vi "rawpower2totalprad.vi"(1 "SampleTime":sgl=0.0032, 3 "width":i32=1, 4 "threshold":dbl=0.00012, 8 "Pre-start time (ms) of\nDAQ":i32=10000, 9 "AddOnTime":sgl=5.0, 10 "samples to exclude":u32=1000, 11 "kbolott_and_volume":dbl[][](array[numeric])=[[1e-05, 1e-05], [9.8364458e-05, 1.8160732], [0.00029863964, 770.25441], [0.00053910452, 1653.5432], [0.00071569496, 2554.7619], [0.00083348142, 3356.1809], [0.00092645429, 4021.9678], [0.00099241932, 4570.4466], [0.0010332482, 4989.6792], [0.0010552469, 5170.4882], [0.0010669981, 5192.5645], [0.001071534, 5152.6222], [0.0010766644, 5109.6704], [0.0010841289, 5094.9972], [0.0010884845, 5078.237], [0.0010888843, 5058.9416], [0.0010882289, 5056.581], [0.0010872861, 5078.1684], [0.0010832221, 5096.5196], [0.0010760805, 5113.7904], [0.0010685167, 5141.4566], [0.0010644166, 5189.7831], [0.0010539441, 5182.7365], [0.0010337779, 5034.6928], [0.00098716411, 4625.8518], [0.00091599422, 4090.3707], [0.00082376071, 3438.9665], [0.00070194108, 2659.5109], [0.00051785958, 1753.3355], [0.00030745544, 937.82125], [0.00014081292, 59.55205], [1e-05, 1e-05], [0.0, 0.0], [0.0, 0.0], [0.0, 0.0], [0.0, 0.0], [0.0, 0.0], [0.0, 0.0], [0.0, 0.0], [0.0, 0.0], [0.0, 0.0], [0.0, 0.0], [0.0, 0.0], [0.0, 0.0], [0.0, 0.0], [0.0, 0.0], [0.0, 0.0], [0.0, 0.0], [0.0019134875, 3474.3085], [0.0020594744, 3690.1455], [0.002175929, 3861.3028], [0.0022530617, 3956.5918], [0.0023492529, 4057.9903], [0.0024581424, 4205.0841], [0.0025383764, 4324.9746], [0.0025876415, 4417.9525], [0.0026676725, 4566.0612], [0.0027635964, 4770.6296], [0.0028188521, 4914.295], [0.0028263806, 4970.0105], [0.0028491244, 5014.7926], [0.0028762033, 5060.279], [0.0028430703, 4969.1072], [0.0027058578, 4592.2853], [0.0019047772, 4936.5706], [0.0023594746, 6388.5028], [0.0025094117, 6336.5413], [0.002569351, 6048.9284], [0.0026367277, 5794.3031], [0.002714522, 5668.1597], [0.0027530637, 5505.217], [0.0027520905, 5312.6378], [0.0027781484, 5183.8321], [0.0028283925, 5165.5044], [0.0028425709, 5118.655], [0.00281436, 5016.5122], [0.0027996491, 4909.784], [0.0027993913, 4845.125], [0.0027603692, 4728.4661], [0.0026886073, 4585.7454], [0.0026437627, 4495.4419], [0.0026242501, 4486.7206], [0.0025685332, 4434.986], [0.0024747416, 4324.8822], [0.0023915919, 4209.8149], [0.002319616, 4111.844], [0.0022042921, 3923.4955], [0.0020485146, 3644.5259], [0.0024033884, 3597.1969], [0.002066694, 2566.1598], [0.0017718795, 1878.4004], [0.0015136288, 1414.3006], [0.0013043692, 1094.5581], [0.0011378765, 882.65731], [0.00097324167, 712.97006], [0.00080739571, 571.52867], [0.0, 0.0], [0.0, 0.0], [0.0, 0.0], [0.0, 0.0], [0.0, 0.0], [0.0, 0.0], [0.0, 0.0], [0.0, 0.0], [0.0, 0.0], [0.0, 0.0], [0.0, 0.0], [0.0, 0.0], [0.0, 0.0], [0.0, 0.0], [0.0, 0.0], [0.0, 0.0], [0.0, 0.0], [0.0, 0.0], [0.0, 0.0], [0.0, 0.0], [0.0, 0.0], [0.0, 0.0], [0.0, 0.0], [0.0, 0.0], [0.0, 0.0], [0.0, 0.0], [0.0, 0.0], [0.0, 0.0], [0.0, 0.0], [0.0, 0.0], [0.0, 0.0], [0.0, 0.0]], 12 "No. of Samples\n[TOA / Sample Rate]":i32=8829, 13 "tau_fact":dbl[](array[numeric])=[0.9942754325698635, 0.9942874264772165, 0.9945323434853295, 0.9944942634351588, 0.9943224506450672, 0.9943408937418631, 0.995821993302933, 0.9945771384409823, 0.9944620036742867, 0.9944762183578384, 0.9939064850392964, 0.9942348416823442, 0.9941481394691951, 0.9939736217416081, 0.9940920651258721, 0.9938858383903332, 0.9946231806379121, 0.9946794273486279, 0.9945386493082798, 0.9945088068622799, 0.9885887214081416, 0.9944821982358365, 0.9942590170035959, 0.9943949158017914, 0.9944259674033434, 0.9942557134338033, 0.9943682303140012, 0.9944129847299683, 0.9937053838258036, 0.9937063363597569, 0.9937961958887874, 0.993777190579244, 0.9967727911662049, 0.9954284436124313, 0.9947198089384633, 0.9947945758851272, 0.992855835614686, 0.9951259961796087, 0.9915396916800793, 0.9938777213378227, 0.9925620075631091, 0.9939808571119726, 0.9953730857234031, 0.9949446485350009, 0.9951693651989406, 0.9938965230094928, 0.9939251148981592, 0.993919756464684, 0.9955634864440348, 0.9965442790473252, 0.9958326248057368, 0.9959297989255841, 0.9946741668106229, 0.9961317432538527, 0.9940816674176194, 0.9956134846505059, 0.994696761237249, 0.9956489327005682, 0.9957202726127232, 0.9952614295331398, 0.9953602706677246, 0.9943075252732968, 0.99446916653835, 0.9944158295695202, 0.9942767772483964, 0.9941050695859821, 0.9944374591927472, 0.9945090337805454, 0.994559907934673, 0.9945848227562215, 0.9948370294812288, 0.9946407805595008, 0.9947163757511401, 0.9944559864420973, 0.994448676943994, 0.9945138262559567, 0.9946225671933909, 0.9946033931105569, 0.9945303195379069, 0.9943576342591244, 0.9939005664775309, 0.993829355141712, 0.9940758603249683, 0.9945212190107237, 0.9945653472775302, 0.9944883825084508, 0.9944285415381326, 0.9969718967619399, 0.9934533430051062, 0.9934476065516122, 0.994137584128452, 0.9939183969854989, 0.9929544573919961, 0.9927976688292449, 0.9926525324439995, 0.9925179780752803, 0.993697881831798, 0.9938832006928247, 0.9939451412935264, 1.0, 0.9934735935885004, 0.9936498588825847, 0.9936377263535082, 0.9938649606619758, 0.9927081189806816, 0.9928561967168806, 0.9930023684194763, 0.9930998249399461, 0.9931265778529161, 0.9931539659381708, 0.9932420399385089, 1.0, 0.9931786270549593, 1.0, 1.0, 1.0, 1.0, 1.0, 1.0, 1.0, 1.0, 1.0, 1.0, 1.0, 1.0, 1.0, 1.0, 1.0], 15 "F_ch":dbl[](array[numeric])=[0.41946313361925236, 0.41267288435379323, 0.4242513967796445, 0.4168638482034789, 0.41940297094410406, 0.41277199910121876, 0.5005048325232518, 0.41804357116097796, 0.4263914266029813, 0.42960951092847915, 0.390161915811526, 0.40903209292753795, 0.4178724636706656, 0.40639561524491535, 0.4168972961680756, 0.4081753936316892, 0.4308482203292378, 0.42985423214074037, 0.4219523533476951, 0.42368590442341997, 0.14968177217291742, 0.4163100359962662, 0.4023134454260441, 0.414083420090156, 0.4104404162383056, 0.40109746288400294, 0.4118376955811143, 0.4106810858926003, 0.4024662767215043, 0.39776761041402614, 0.39988820944073605, 0.3960937680653605, 0.39631376832177734, 0.46359628762328325, 0.4330664870101722, 0.42809053434855326, 0.3663794753981563, 0.4515112216941263, 0.32097119732923274, 0.38596625816052027, 0.35592992953912717, 0.3967614343688723, 0.4769395376117402, 0.4603968175127216, 0.45645057575669823, 0.40983050619896044, 0.41762784967370237, 0.4195235233012393, 0.4869668482151368, 0.5451176818983113, 0.4981002466254468, 0.5025919311483945, 0.4408139623514431, 0.5086015118188133, 0.4212525350361159, 0.489548299707763, 0.44280968589083947, 0.4733195391787026, 0.48968023906864, 0.46123705868954207, 0.48585880384966634, 0.43109305912935353, 0.42964432162914334, 0.43379373132681903, 0.4103150055137274, 0.41637546628976474, 0.4240718501347476, 0.43097541489804153, 0.42854727670203413, 0.43071258286250785, 0.4538231011436137, 0.43842591900842043, 0.44773109787963017, 0.43813274820972226, 0.4477786314686775, 0.43083627933543217, 0.4448007784686704, 0.4463858689900978, 0.44471759411780265, 0.43905527786878207, 0.40988850494900064, 0.4042286595549796, 0.4210125779131261, 0.42523385782519874, 0.43930897084124976, 0.4317134422486339, 0.42503793161390413, 0.5866703715028357, 0.3713420175081803, 0.3729221791024955, 0.421847369908469, 0.4038171530405619, 0.3723947010396081, 0.36905241334809796, 0.365027355646126, 0.35883096352560634, 0.38453723852279414, 0.3908590433215044, 0.3942344477458136, -inf, 0.37872098293573886, 0.38823921546406664, 0.38647066465095736, 0.4010630278464888, 0.3699009376238012, 0.37440275442115767, 0.378492662918438, 0.37713022559389764, 0.375270284145916, 0.37421667685537685, 0.3729410641899398, inf, 0.367989869633843, -inf, -inf, -inf, -inf, -inf, inf, -inf, -inf, -inf, -inf, inf, inf, inf, -inf, inf], 17 "TauM":dbl[](array[numeric])=[0.10247326273143675, 0.10385139756960429, 0.10373232144795708, 0.10311875959492485, 0.1040387663981229, 0.1046650716638566, 0.10127197371489062, 0.10433939668939028, 0.09961240211936159, 0.10113688577012743, 0.09820100289764892, 0.10095901838579123, 0.10145991266213297, 0.10133898562095205, 0.10130127833216106, 0.09956334469474118, 0.10358378126227558, 0.1033444650149854, 0.10368122845865657, 0.1024629201687842, 0.10726822954303422, 0.10182022977214773, 0.10234341921814957, 0.10309722284273504, 0.1042952251760315, 0.10251907726247211, 0.10376892017069193, 0.10390613836510422, 0.10393962152806514, 0.10278682866750612, 0.1029066416867304, 0.102809145991027, 0.10885131092677319, 0.09862497604372066, 0.10044854636642224, 0.1011397796494332, 0.10002902352125999, 0.09964990042145319, 0.10015936689391987, 0.10006472096945454, 0.09839726301474191, 0.0989699304142558, 0.1002391552504395, 0.10013350870556857, 0.10080436633835735, 0.09779852218595043, 0.09742571115181148, 0.09710433370493086, 0.10444501045101653, 0.1003366401072974, 0.10437315691375147, 0.10384291417884778, 0.10124021541103015, 0.10550745222701648, 0.1035137865735804, 0.10352859881892808, 0.1012417667717822, 0.1059159267079176, 0.10317764912629153, 0.10345604684447908, 0.1049337703539443, 0.10334536377187596, 0.1011439242990685, 0.10281039287381427, 0.10222071286894058, 0.10128943771143158, 0.10126644136767568, 0.10213051552429299, 0.10166794227392674, 0.10164755793457868, 0.10028065773083647, 0.1039274155284877, 0.10062166309448936, 0.10100667896022858, 0.10122793031614634, 0.1020869722455638, 0.10086834901007827, 0.10107073060568635, 0.10100593381229647, 0.1013148799331511, 0.10336010473304796, 0.104020047148851, 0.10319519163947051, 0.1023647743297228, 0.10121262984849082, 0.10131571623308212, 0.10129251089534078, 0.10505043416568437, 0.10066202738446095, 0.10001990246198598, 0.10320829246582676, 0.10342094956544687, 0.10072458787609094, 0.10113661913958252, 0.10213104126735983, 0.10141193462449195, 0.10097352152629059, 0.1005352087055146, 0.09991412160243203, 0.0, 0.09971962753116924, 0.10038664478845472, 0.0996831725438015, 0.0987164166127979, 0.10070743969491262, 0.10083769719722958, 0.09991070137880578, 0.09976037466686079, 0.09975950391708734, 0.0997863315853558, 0.09952725945462769, 0.0, 0.09982037400508142, 0.0, 0.0, 0.0, 0.0, 0.0, 0.0, 0.0, 0.0, 0.0, 0.0, 0.0, 0.0, 0.0, 0.0, 0.0] format="%10.4f", 19 "RawArray":sgl[][](array[numeric])=array128x7829[1002112 elements]) -> (16 "corrected voltage array":dbl[][](array[numeric]), 18 "AdjustedPower":dbl[][](array[numeric]), 22 "P_rad HBC [MW]":dbl[](array[numeric]), 23 "P_rad VBC [MW]":dbl[](array[numeric]))   [LabVIEW 2014]
uses:
  <vilib>/Analysis/baseanly.llb/Mean (DBL).vi
  <vilib>/Analysis/3filter.llb/FIR Filter (DBL).vi
  <vilib>/Analysis/NI_AALBase.lvlib
  <vilib>/Analysis/NI_AALPro.lvlib
  <vilib>/Analysis/3filter.llb/Savitzky-Golay Filter (DBL).vi
panel:
  out "Time":dbl[](array[numeric])
  out "ECRH OFF SAMPLE":i64
  out "empty sample array":dbl[](array[numeric])
  out "ECRH ON SAMPLE":i64=2156
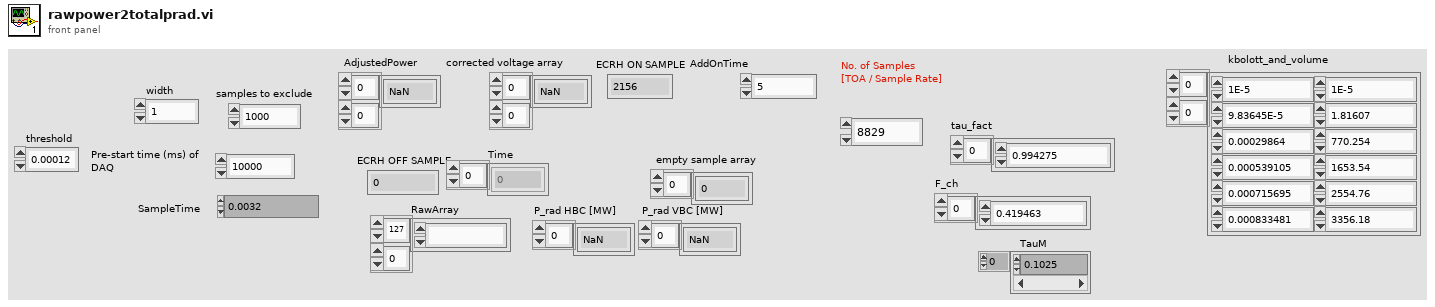
[diagram p1: front panel]
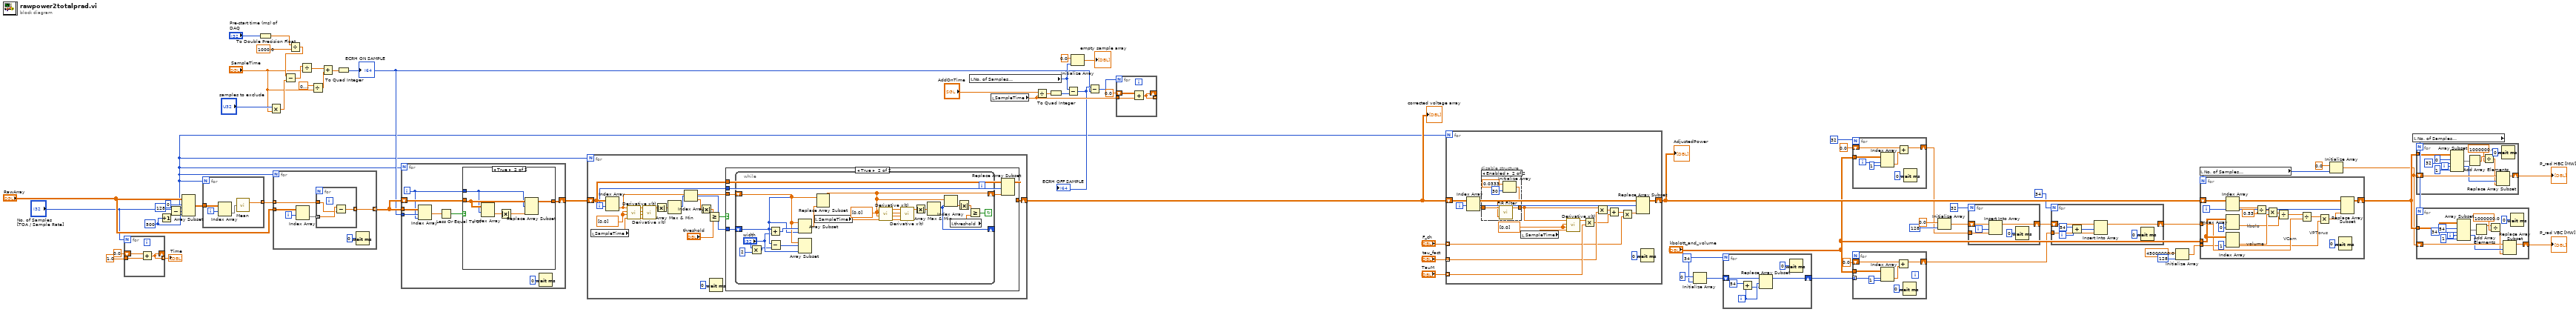
[diagram p0: block diagram]
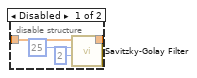
[diagram p3: hidden frame]
diagram:
  w36 = 34
  w2 = 128 ("length")
  w11 = 500 ("y")
  n1 = for {
    N: "No. of Samples\n[TOA / Sample Rate]" -> [_]
    tunnel: [w72] -> w4 mode=indexing
    shift-right: [w72] -> _
    shift-left: 0.0 -> [w71]
    tunnel: sgl 1.0 ("SampleTime") -> [w70]
    n2 = Add(x=w71, y=w70) -> (x+y=w72:dbl)
  }
  "Time" <- w4
  n3 = Increment(x=w11) -> (x+1=w10:i32)
  n4 = Subtract(x="No. of Samples\n[TOA / Sample Rate]", y=w10) -> (x-y=w69:i32)
  n5 = Array Subset(array="RawArray", index (row)=0 ("index"), length (row)=w2, index (col)=w69, length (col)=w11) -> (w67:sgl[][])
  n6 = for {
    N: w2 -> [_]
    tunnel: w67 -> [w74]
    tunnel: [w76] -> w66 mode=indexing
    i -> [w73]
    n7 = Index Array(array=w74, index (row)=w73) -> (element=w75:sgl[])  [unwired: 1 in]
    n8 = call-poly <vilib>:"Mean.vi"("X"=w75) -> ("mean"=w76:dbl)  [unwired: 1 out]
  }
  n9 = To Double Precision Float(number="Pre-start time (ms) of\nDAQ") -> (double precision float=w61:dbl)
  n10 = Multiply(x="samples to exclude", y="SampleTime") -> (x*y=w63:sgl)
  n11 = for {
    N: w2 -> [_]
    tunnel: w66 -> [w80] mode=indexing
    tunnel: "RawArray" -> [w82]
    tunnel: [w78] -> w53 mode=indexing
    i -> [w81]
    n12 = Index Array(array=w82, index (row)=w81) -> (element=w79:sgl[])  [unwired: 1 in]
    n13 = for {
      tunnel: w79 -> [w85] mode=indexing
      tunnel: w80 -> [w84]
      tunnel: [w83] -> w78 mode=indexing
      n14 = Subtract(x=w85, y=w84) -> (x-y=w83:dbl)
    }
    n15 = Wait (ms)(milliseconds to wait=u32 0) -> ()  [unwired: 1 out]
  }
  n16 = Divide(x=w61, y=1000.0) -> (x/y=w59:dbl)
  n17 = Subtract(x=w59, y=w63) -> (x-y=w62:dbl)
  n18 = Divide(x=w62, y="SampleTime") -> (x/y=w58:dbl)
  n19 = Divide(x=sgl 0.1, y="SampleTime") -> (x/y=w54:sgl)
  n20 = Add(x=w58, y=w54) -> (x+y=w57:dbl)
  n21 = To Quad Integer(1:w57) -> (0:w3:i64)
  "ECRH ON SAMPLE" <- w3
  n22 = for {
    N: w2 -> [_]
    tunnel: w53 -> [w93]
    tunnel: w3 -> [w92]
    shift-right: [w87] -> w8
    shift-left: w53 -> [w89]
    i -> [w88]
    n23 = Index Array(array=w93, index (row)=w92, index (col)=w88) -> (element=w91:dbl)
    n24 = Less Or Equal To 0?(x=w91) -> (x <= 0?=w90:bool)
    n25 = case shown="True" w90 {
      tunnel: w89 -> [w94 w99]
      tunnel: w88 -> [_ w98]
      tunnel: [w94 w97] -> w87
      frame False {
      }
      frame True {
        n26 = Index Array(array=w99, index (row)=w98) -> (element=w96:dbl[])  [unwired: 1 in]
        n27 = Absolute Value(x=w96) -> (abs(x)=w95:dbl[])
        n28 = Replace Array Subset(array=w99, new element=w95, index (row)=w98) -> (w97:dbl[][])  [unwired: 1 in]
      }
    }
    n29 = Wait (ms)(milliseconds to wait=u32 0) -> ()  [unwired: 1 out]
  }
  n30 = for {
    N: w2 -> [_]
    shift-right: [w101] -> w7
    shift-left: w8 -> [w108]
    i -> [w100]
    w113 = dbl[] [0.0] ("Initial Condition")
    n31 = local read "SampleTime"() -> (w112:sgl)
    n32 = Index Array(array=w108, index (row)=w100) -> (element=w102:dbl[])  [unwired: 1 in]
    n33 = call <vilib>:"Derivative x(t).vi"("dt"=w112, "Final Condition"=w113, "Initial Condition"=w113, "X"=w102) -> ("dX/dt"=w114:dbl[])  [unwired: 6 in, 1 out]
    n34 = call <vilib>:"Derivative x(t).vi"("dt"=w112, "Final Condition"=w113, "Initial Condition"=w113, "X"=w114) -> ("dX/dt"=w111:dbl[])  [unwired: 6 in, 1 out]
    n35 = Absolute Value(x=w111) -> (abs(x)=w103:dbl[])
    n36 = Array Max & Min(array=w103) -> (max index (indices)=w107:i32)  [unwired: 3 out]
    n37 = Index Array(array=w102, index=w107) -> (element=w106:dbl)
    n38 = Absolute Value(x=w106) -> (abs(x)=w105:dbl)
    n39 = Greater Or Equal?(x=w105, y="threshold") -> (x >= y?=w109:bool)
    n40 = Wait (ms)(milliseconds to wait=u32 0) -> ()  [unwired: 1 out]
    n41 = case shown="True" w109 {
      tunnel: w102 -> [_ w121]
      tunnel: w100 -> [_ w116]
      tunnel: w108 -> [w115 w119]
      tunnel: [w115 w118] -> w101
      tunnel: w107 -> [_ w120]
      frame False {
      }
      frame True {
        n42 = while {
          shift-right: [w122] -> w117
          shift-left: w121 -> [w137]
          shift-right: [w126] -> _
          shift-left: w120 -> [w136]
          stop <- w127 continue-if-true
          w134 = dbl[] [0.0] ("Initial Condition")
          n43 = Multiply(x="width", y=2) -> (x*y=w123:i32)
          n44 = Add(x=w136, y="width") -> (x+y=w138:i32)
          n45 = Subtract(x=w136, y=w123) -> (x-y=w139:i32)
          n46 = Array Subset(array=w137, index=w138, length=w136) -> (w135:dbl[])
          n47 = Array Subset(array=w137, index=w139, length="width") -> ()  [unwired: 1 out]
          n48 = local read "SampleTime"() -> (w140:sgl)
          n49 = Replace Array Subset(array=w137, new element=w135, index=w136) -> (w122:dbl[])
          n50 = call <vilib>:"Derivative x(t).vi"("dt"=w140, "Final Condition"=w134, "Initial Condition"=w134, "X"=w122) -> ("dX/dt"=w133:dbl[])  [unwired: 6 in, 1 out]
          n51 = call <vilib>:"Derivative x(t).vi"("dt"=w140, "Final Condition"=w134, "Initial Condition"=w134, "X"=w133) -> ("dX/dt"=w131:dbl[])  [unwired: 6 in, 1 out]
          n52 = Absolute Value(x=w131) -> (abs(x)=w132:dbl[])
          n53 = Array Max & Min(array=w132) -> (max index (indices)=w126:i32)  [unwired: 3 out]
          n54 = Index Array(array=w122, index=w126) -> (element=w130:dbl)
          n55 = local read "threshold"() -> (w128:dbl)
          n56 = Absolute Value(x=w130) -> (abs(x)=w129:dbl)
          n57 = Greater Or Equal?(x=w129, y=w128) -> (x >= y?=w127:bool)
        }
        n58 = Replace Array Subset(array=w119, new element=w117, index (row)=w116) -> (w118:dbl[][])  [unwired: 1 in]
      }
    }
  }
  "corrected voltage array" <- w7
  n59 = local read "No. of Samples\n[TOA / Sample Rate]"() -> (w44:i32)
  n60 = local read "SampleTime"() -> (w48:sgl)
  n61 = Divide(x="AddOnTime", y=w48) -> (x/y=w51:sgl)
  n62 = To Quad Integer(1:w51) -> (0:w50:i64)
  n63 = Subtract(x=w44, y=w50) -> (x-y=w46:i64)
  "ECRH OFF SAMPLE" <- w46
  n64 = Initialize Array(0.0 ("element"), w44) -> (→"empty sample array":dbl[])
  n65 = Subtract(x=w46, y=w3) -> (x-y=w47:i64)
  n66 = for {
    N: w47 -> [_]
    tunnel: [w143] -> _ mode=indexing
    shift-right: [w143] -> _
    shift-left: 0.0 -> [w142]
    tunnel: w48 -> [w141]
    n67 = Add(x=w142, y=w141) -> (x+y=w143:dbl)
  }
  n68 = for {
    N: w2 -> [_]
    shift-right: [w157] -> w39
    shift-left: w7 -> [w156]
    tunnel: "F_ch" -> [w149] mode=indexing
    tunnel: "tau_fact" -> [w153] mode=indexing
    tunnel: "TauM" -> [w154] mode=indexing
    i -> [w155]
    w159 = dbl[] [0.0] ("Initial Condition")
    n69 = Index Array(array=w156, index (row)=w155) -> (element=w147:dbl[])  [unwired: 1 in]
    n70 = disable-structure shown="Enabled" {
      disable-tunnel: w147 -> [w161 w167]
      disable-tunnel: [w160 w166] -> w145
      frame Disabled {
        n71 = call-poly <vilib>:"Savitzky-Golay Filter.vi"("polynomial order"=2, "side points"=25, "X"=w161) -> ("Filtered X"=w160:dbl[])  [unwired: 7 in, 1 out]
      }
      frame Enabled {
        n72 = Initialize Array(0.0333 ("element"), 30 ("dimension size")) -> (w164:dbl[])
        n73 = call-poly <vilib>:"FIR Filter.vi"("FIR Coefficients"=w164, "X"=w167) -> ("Filtered X"=w166:dbl[])  [unwired: 2 in, 1 out]
      }
    }
    n74 = local read "SampleTime"() -> (w158:sgl)
    n75 = call <vilib>:"Derivative x(t).vi"("dt"=w158, "Final Condition"=w159, "Initial Condition"=w159, "X"=w145) -> ("dX/dt"=w146:dbl[])  [unwired: 6 in, 1 out]
    n76 = Multiply(x=w146, y=w154) -> (x*y=w151:dbl[])
    n77 = Multiply(x=w145, y=w153) -> (x*y=w152:dbl[])
    n78 = Add(x=w152, y=w151) -> (x+y=w150:dbl[])
    n79 = Multiply(x=w150, y=w149) -> (x*y=w148:dbl[])
    n80 = Replace Array Subset(array=w156, new element=w148, index (row)=w155) -> (w157:dbl[][])  [unwired: 1 in]
    n81 = Wait (ms)(milliseconds to wait=u32 0) -> ()  [unwired: 1 out]
  }
  "AdjustedPower" <- w39
  n82 = Initialize Array(0, w36) -> (w35:i32[])
  n83 = for {
    N: w36 -> [_]
    shift-right: [w170] -> w34
    shift-left: w35 -> [w171]
    i -> [w174]
    n84 = Add(x=54, y=w174) -> (x+y=w172:i32)
    n85 = Replace Array Subset(array=w171, new element=w172, index=w174) -> (w170:i32[])
    n86 = Wait (ms)(milliseconds to wait=u32 0) -> ()  [unwired: 1 out]
  }
  n87 = for {
    tunnel: "kbolott_and_volume" -> [w181]
    shift-right: [w177] -> w25
    shift-left: 0.0 ("V_Cam") -> [w178]
    tunnel: w34 -> [w176] mode=indexing
    n88 = Index Array(array=w181, index (row)=w176, index (col)=1 ("disabled index (col)")) -> (element=w180:dbl)
    n89 = Add(x=w178, y=w180) -> (x+y=w177:dbl)
    n90 = Wait (ms)(milliseconds to wait=u32 0) -> ()  [unwired: 1 out]
  }
  n91 = for {
    N: 32 -> [_]
    tunnel: "kbolott_and_volume" -> [w188]
    shift-right: [w184] -> w27
    shift-left: 0.0 ("V_Cam") -> [w185]
    i -> [w183]
    n92 = Index Array(array=w188, index (row)=w183, index (col)=1 ("disabled index (col)")) -> (element=w187:dbl)
    n93 = Add(x=w185, y=w187) -> (x+y=w184:dbl)
    n94 = Wait (ms)(milliseconds to wait=u32 0) -> ()  [unwired: 1 out]
  }
  n95 = Initialize Array(0.0 ("element"), 128 ("dimension size")) -> (w29:dbl[])
  n96 = for {
    N: 32 -> [_]
    shift-right: [w190] -> w26
    shift-left: w29 -> [w193]
    tunnel: w27 -> [w191]
    i -> [w192]
    n97 = Insert Into Array(array=w193, index=w192, new element=w191) -> (w190:dbl[])
    n98 = Wait (ms)(milliseconds to wait=u32 0) -> ()  [unwired: 1 out]
  }
  n99 = for {
    N: 34 -> [_]
    shift-right: [w195] -> w24
    shift-left: w26 -> [w198]
    tunnel: w25 -> [w196]
    i -> [w199]
    n100 = Add(x=54, y=w199) -> (x+y=w197:i32)
    n101 = Insert Into Array(array=w198, index=w197, new element=w196) -> (w195:dbl[])
    n102 = Wait (ms)(milliseconds to wait=u32 0) -> ()  [unwired: 1 out]
  }
  n103 = Initialize Array(45000000.0 ("element"), 128 ("dimension size")) -> (w21:dbl[])
  n104 = local read "No. of Samples\n[TOA / Sample Rate]"() -> (w18:i32)
  n105 = for {
    N: w18 -> [_]
    tunnel: "kbolott_and_volume" -> [w218]
    tunnel: w24 -> [w208]
    tunnel: w21 -> [w206]
    shift-right: [w202] -> w20
    shift-left: w39 -> [w205]
    i -> [w204]
    # "VPTorus"
    # "VCam"
    # "kbolo"
    # "volume"
    n106 = Index Array(array=w205, index (col)=w204) -> (element=w215:dbl[])  [unwired: 1 in]
    n107 = Index Array(array=w218, index (col)=0 ("disabled index (col)")) -> (element=w210:dbl[])  [unwired: 1 in]
    n108 = Index Array(array=w218, index (col)=1 ("disabled index (col)")) -> (element=w212:dbl[])  [unwired: 1 in]
    n109 = Divide(x=w215, y=0.53) -> (x/y=w213:dbl[])
    n110 = Multiply(x=w213, y=w212) -> (x*y=w211:dbl[])
    n111 = Divide(x=w211, y=w210) -> (x/y=w209:dbl[])
    n112 = Divide(x=w209, y=w208) -> (x/y=w207:dbl[])
    n113 = Multiply(x=w207, y=w206) -> (x*y=w203:dbl[])
    n114 = Wait (ms)(milliseconds to wait=u32 0) -> ()  [unwired: 1 out]
    n115 = Replace Array Subset(array=w205, new element=w203, index (col)=w204) -> (w202:dbl[][])  [unwired: 1 in]
  }
  n116 = Initialize Array(0.0 ("element"), w18) -> (w17:dbl[])
  n117 = local read "No. of Samples\n[TOA / Sample Rate]"() -> (w16:i32)
  n118 = for {
    N: w16 -> [_]
    tunnel: w20 -> [w230]
    shift-right: [w223] -> w12
    shift-left: w17 -> [w225]
    i -> [w224]
    n119 = Array Subset(array=w230, index (row)=0 ("index"), length (row)=32 ("length"), index (col)=w224, length (col)=1 ("length")) -> (w226:dbl[][])
    n120 = Add Array Elements(numeric array=w226) -> (sum=w221:dbl)
    n121 = Divide(x=w221, y=1000000.0 ("x")) -> (x/y=w222:dbl)
    n122 = Replace Array Subset(array=w225, new element=w222, index=w224) -> (w223:dbl[])
    n123 = Wait (ms)(milliseconds to wait=u32 0) -> ()  [unwired: 1 out]
  }
  "P_rad HBC [MW]" <- w12
  n124 = for {
    N: w16 -> [_]
    tunnel: w20 -> [w236]
    shift-right: [w237] -> w13
    shift-left: w17 -> [w238]
    i -> [w235]
    n125 = Array Subset(array=w236, index (row)=54 ("index"), length (row)=34 ("length"), index (col)=w235, length (col)=1 ("length")) -> (w239:dbl[][])
    n126 = Add Array Elements(numeric array=w239) -> (sum=w232:dbl)
    n127 = Divide(x=w232, y=1000000.0 ("x")) -> (x/y=w234:dbl)
    n128 = Replace Array Subset(array=w238, new element=w234, index=w235) -> (w237:dbl[])
    n129 = Wait (ms)(milliseconds to wait=u32 0) -> ()  [unwired: 1 out]
  }
  "P_rad VBC [MW]" <- w13
